vi "Configure_Trigger_Gate.vi"(8 "error in (no error)":errorcluster, 9 "ON/OFF TRIGGER":bool, 11 "VISA resource name":refnum<visa-resource-name>) -> (0 "error out":errorcluster)   [LabVIEW 2021]
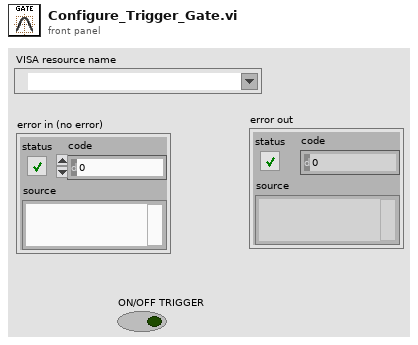
[diagram p1: front panel]
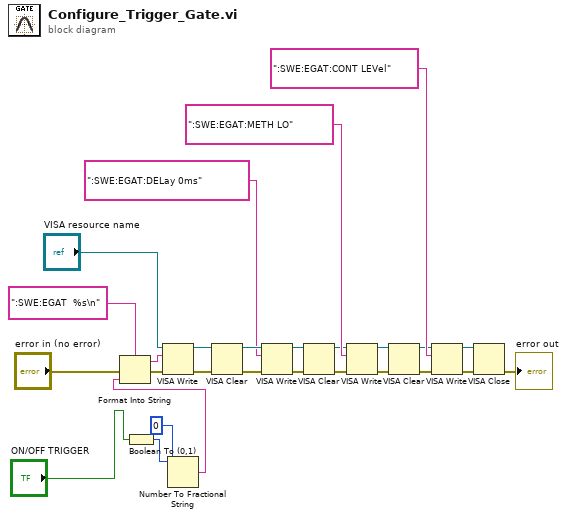
[diagram p0: block diagram]
diagram:
  n1 = Boolean To (0,1)(Boolean="ON/OFF TRIGGER") -> (0, 1=w3:i16)
  n2 = Number To Fractional String(number=w3, precision (6)=i16 0) -> (F-format string=w1:string)  [unwired: 2 in]
  n3 = Format Into String(format string=":SWE:EGAT  %s\n" ("string"), error in="error in (no error)", w1) -> (resulting string=w7:string, error out=w5:errorcluster)  [unwired: 1 in]
  n4 = VISA Write(VISA resource name="VISA resource name", write buffer=w7, error in (no error)=w5) -> (VISA resource name out=w25:refnum<visa-resource-name>, error out=w24:errorcluster)  [unwired: 1 out]
  n5 = VISA Clear(VISA resource name=w25, error in (no error)=w24) -> (VISA resource name out=w23:refnum<visa-resource-name>, error out=w22:errorcluster)
  n6 = VISA Write(VISA resource name=w23, write buffer=":SWE:EGAT:DELay 0ms" ("string"), error in (no error)=w22) -> (VISA resource name out=w19:refnum<visa-resource-name>, error out=w18:errorcluster)  [unwired: 1 out]
  n7 = VISA Clear(VISA resource name=w19, error in (no error)=w18) -> (VISA resource name out=w15:refnum<visa-resource-name>, error out=w16:errorcluster)
  n8 = VISA Write(VISA resource name=w15, write buffer=":SWE:EGAT:METH LO" ("string"), error in (no error)=w16) -> (VISA resource name out=w14:refnum<visa-resource-name>, error out=w13:errorcluster)  [unwired: 1 out]
  n9 = VISA Clear(VISA resource name=w14, error in (no error)=w13) -> (VISA resource name out=w12:refnum<visa-resource-name>, error out=w11:errorcluster)
  n10 = VISA Write(VISA resource name=w12, write buffer=":SWE:EGAT:CONT LEVel" ("string"), error in (no error)=w11) -> (VISA resource name out=w10:refnum<visa-resource-name>, error out=w9:errorcluster)  [unwired: 1 out]
  n11 = VISA Close(VISA resource name=w10, error in (no error)=w9) -> (error out=→"error out":errorcluster)
